vi "HideFromMenu.vi"(8 "error in":errorcluster, 9 "Menu hierarchy in":string[](array[string]), 11 "NodePtr":u64) -> (0 "error out":errorcluster, 1 "Menu hierarchy out":string[](array[string]), 3 "Action":enum16{"Enable", "Disable", "Hide"}(ring))   [LabVIEW 2019, in "SLSC EDS System Explorer.lvlib"]
uses:
  SLSC EDS System Explorer.lvlib
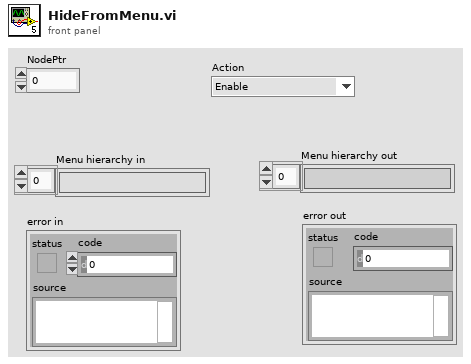
[diagram p1: front panel]
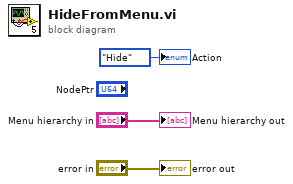
[diagram p0: block diagram]
diagram:
  "error out" <- "error in"
  "Action" <- enum16{"Enable", "Disable", "Hide"}."Hide" ("Action")
  "Menu hierarchy out" <- "Menu hierarchy in"
